vi "RT Main.vi"() -> ()   [LabVIEW 2014]
uses:
  <vilib>/NI/cRIO Wfm/cRIO Wfm.lvlib
  <vilib>/NI/cRIO Wfm/AcqRead(Wfm).vi
  <vilib>/rvi/interface/nirviOpenFPGA/nirviOpenFPGA.xnode
  <vilib>/rvi/interface/nirviMethod/nirviMethod.xnode
  <vilib>/FPGAPlugInAG/Dynamic/niLvFpga_Reset_Dynamic.vi
  <vilib>/FPGAPlugInAG/Dynamic/niLvFpga_Run_Dynamic.vi
  <vilib>/rvi/interface/nirviCloseFPGA/nirviCloseFPGA.xnode
  Perforce/dev-iknox/Sales/users/iknox/FPGA Main_SPI API.vi
  <vilib>/FPGAPlugInAG/Dynamic/niLvFpga_Close_Dynamic.vi
  <vilib>/NI/cRIO Wfm/ChannelConfig.ctl
panel:
  in  "stop":bool
  out "Waveform Chart":waveform(sgl)[](graph)
  in  "Sample Rate":u32=1000
  in  "Samples per Channel":i32=1000
  in  "Sample Mode":enum16{"Finite Samples", "Continuous Samples"}(ring)=enum."Continuous Samples"
  in  "Channel Info":T1=[{"Channel Name"="Untitled", "Sensitivity mV_EU"=1000.0, "EU"="V", "dB Ref EU"=1.0}, {"Channel Name"="Untitled", "Sensitivity mV_EU"=1000.0, "EU"="V", "dB Ref EU"=1.0}, {"Channel Name"="Untitled", "Sensitivity mV_EU"=1000.0, "EU"="V", "dB Ref EU"=1.0}, {"Channel Name"="Untitled", "Sensitivity mV_EU"=1000.0, "EU"="V", "dB Ref EU"=1.0}] {"dB Ref EU" format="%#.2p"; "Sensitivity mV_EU" format="%.2f"}
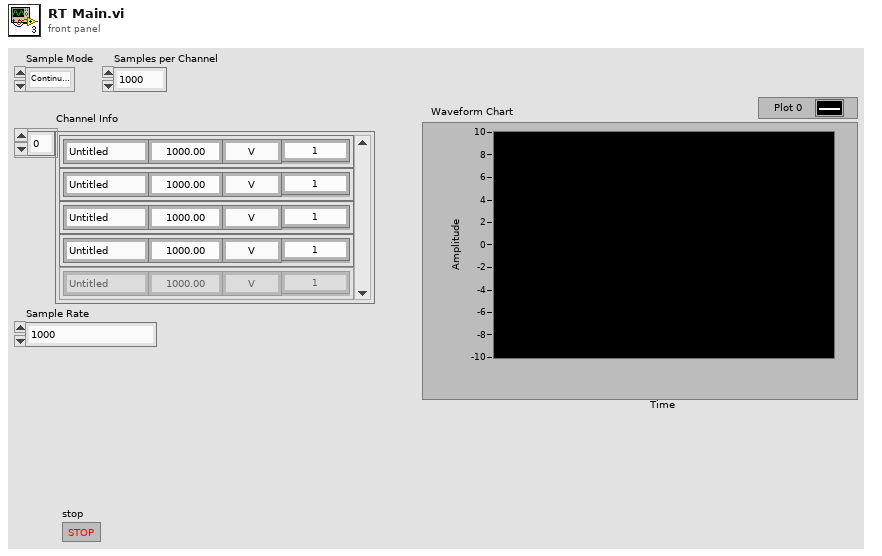
[diagram p1: front panel]
types:
  T1 = typedef "cRIO Wfm.lvlib/ChannelConfig.ctl" = cluster{"Channel Name":string, "Sensitivity mV_EU":dbl, "EU":string, "dB Ref EU":dbl}[]
  T2 = typedef "cRIO Wfm.lvlib/SamplingInfo.ctl" = cluster{"Number of Channels":i32, "Actual Samp Rate":dbl, "Chan Name Array":string[], "EU Chan Array":string[], "dB Ref Chan Array":dbl[]}
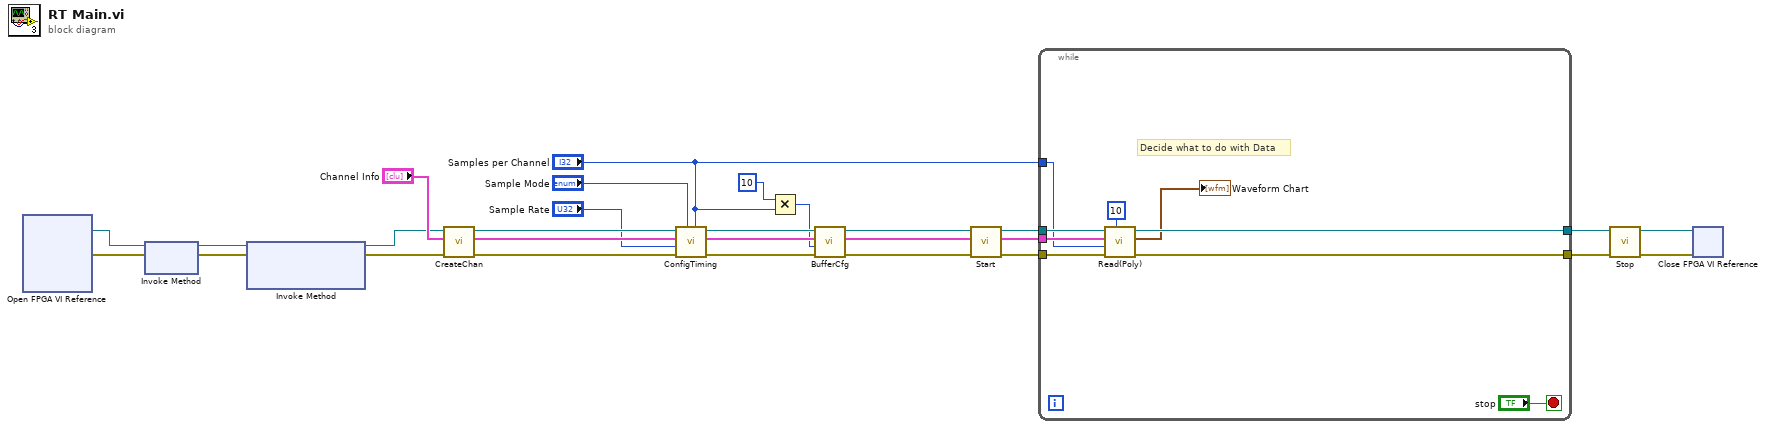
[diagram p0: block diagram]
diagram:
  n1 = xnode "Open FPGA VI Reference"() -> ("FPGA VI Reference Out"=w7:refnum<k20>, "error out"=w8:errorcluster)  [unwired: 2 in]
  n2 = xnode "Invoke Method"("FPGA VI Reference In"=w7, "error in"=w8) -> ("FPGA VI Reference Out"=w6:refnum<k20>, "error out"=w3:errorcluster)
  n3 = xnode "Invoke Method"("FPGA VI Reference In"=w6, "error in"=w3) -> ("FPGA VI Reference Out"=w5:refnum<k20>, "error out"=w4:errorcluster)  [unwired: 1 in]
  n4 = call <vilib>:"CreateChan.vi"("error in"=w4, "Channel Info"="Channel Info", "Dynamic FPGA Ref"=w5) -> ("error out"=w16:errorcluster, "Sampling Info"=w22:T2, "Dynamic FPGA Ref Out"=w28:refnum<k20>)  [unwired: 6 in]
  n5 = call <vilib>:"ConfigTiming.vi"("Samples per Channel"="Samples per Channel", "Sample Mode"="Sample Mode", "error in"=w16, "Sample Rate"="Sample Rate", "Sampling Info In"=w22, "Dynamic FPGA Ref"=w28) -> ("error out"=w15:errorcluster, "Sampling Info Out"=w23:T2, "Dynamic FPGA Ref Out"=w27:refnum<k20>)  [unwired: 2 in, 1 out]
  n6 = Multiply(x=10, y="Samples per Channel") -> (x*y=w18:i32)
  n7 = call <vilib>:"BufferCfg.vi"("error in"=w15, "Buffer Size [Samps per Chan]"=w18, "Sampling Info In"=w23, "Dynamic FPGA Ref"=w27) -> ("error out"=w14:errorcluster, "Sampling Info Out"=w21:T2, "Dynamic FPGA Ref Out"=w26:refnum<k20>)  [unwired: 4 in, 1 out]
  n8 = call <vilib>:"Start.vi"("error in"=w14, "Sampling Info In"=w21, "Dynamic FPGA Ref"=w26) -> ("error out"=w13:errorcluster, "Sampling Info Out"=w12:T2, "Dynamic FPGA Ref Out"=w17:refnum<k20>)  [unwired: 6 in]
  n9 = while {
    tunnel: w17 -> [w37]
    tunnel: w13 -> [w36]
    tunnel: w12 -> [w35]
    tunnel: "Samples per Channel" -> [w33]
    tunnel: [w32] -> w10
    tunnel: [w31] -> w9
    stop <- "stop" stop-if-true
    # "Decide what to do with Data"
    n10 = call-poly <vilib>:"Read(Poly).vi"("Poll Time (ms)"=u32 10, "error in"=w36, "Samps Read per Chan"=w33, "Sampling Info"=w35, "Dynamic FPGA Ref"=w37) -> ("error out"=w31:errorcluster, "Wfm Data"=→"Waveform Chart":waveform(sgl)[], "Dynamic FPGA Ref Out"=w32:refnum<k20>)  [unwired: 3 in, 1 out]
  }
  n11 = call <vilib>:"Stop.vi"("error in"=w9, "Dynamic FPGA Ref"=w10) -> ("error out"=w1:errorcluster, "Dynamic FPGA Ref Out"=w2:refnum<k20>)  [unwired: 8 in]
  n12 = xnode "Close FPGA VI Reference"("FPGA VI Reference In"=w2, "error in"=w1) -> ()  [unwired: 1 out]
